vi "CheckMatchesWorking.vi"(11 "Последен тираж":i64[](array[numeric])) -> (0 "?":i64[][](array[numeric]), 1 "Съвпадения":i32[](array[numeric]), 2 "Залози":i32[][](array[numeric]), 4 "file path (dialog if empty)":path=path "/Users/blagojnikolov/Desktop/@tmp/checkRes.txt")   [LabVIEW 2023]
uses:
  <vilib>/Utility/file.llb/Read Delimited Spreadsheet (I64).vi
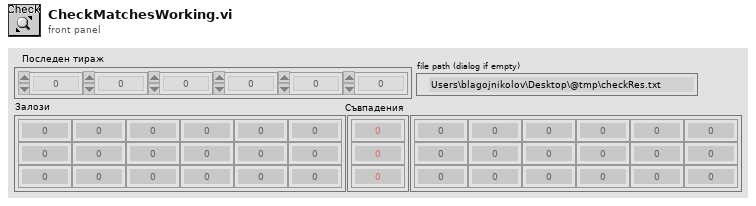
[diagram p1: front panel]
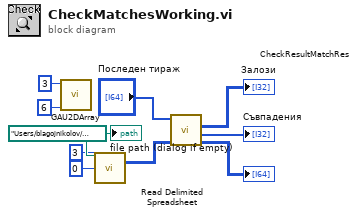
[diagram p0: block diagram]
diagram:
  w4 = path "/Users/blagojnikolov/Desktop/@tmp/checkRes.txt" ("file path (dialog if empty)")
  n1 = call "GAU2DArray.vi"("Colums"=6, "Rows"=3) -> ()  [unwired: 7 in, 3 out]
  n2 = call-poly <vilib>:"Read Delimited Spreadsheet.vi"("file path (dialog if empty)"=w4, "number of rows (all:-1)"=3, "start of read offset (chars.:0)"=0) -> ("all rows"=w3:i64[][])  [unwired: 7 in, 5 out]
  n3 = call "CheckResultMatchRes.vi"("Your Suppose"=w3, "Last Draw"="Последен тираж") -> ("Matches array"=→"?":i64[][], "Matches"=→"Съвпадения":i32[], "Your Suppose"=→"Залози":i64[][])  [unwired: 6 in, 1 out]
  "file path (dialog if empty)" <- w4
